vi "CompareData.vi"(1 "Que Name":string, 2 "Data input":string) -> (0 "Same as before":bool)   [LabVIEW 2011]
doc: "Will compare New data with Old Data where the New data is the current Data input and the Old data is the previous Data input."
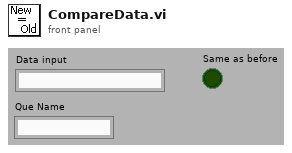
[diagram p1: front panel]
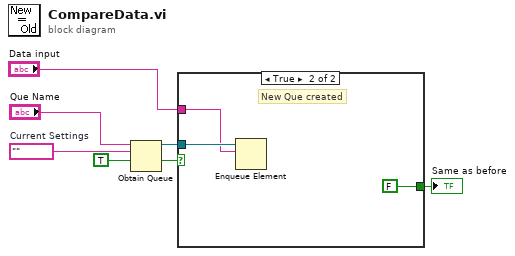
[diagram p0: block diagram]
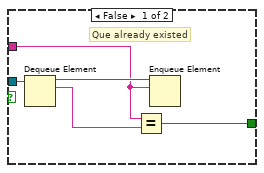
[diagram p2: hidden frame]
diagram:
  w5 = ""  # Current Settings
  n1 = Obtain Queue(name (unnamed)="Que Name", element data type=w5, create if not found? (T)=TRUE) -> (queue out=w6:refnum<queue>, created new?=w4:bool)  [unwired: 2 in, 1 out]
  n2 = case shown="True" w4 {
    tunnel: w6 -> [w12 w15]
    tunnel: "Data input" -> [w9 w14]
    tunnel: [w8 FALSE] -> w2
    frame False {
      # "Que already existed"
      n3 = Dequeue Element(queue=w12) -> (queue out=w11:refnum<queue>, element=w10:string)  [unwired: 2 in, 2 out]
      n4 = Equal?(x=w9, y=w10) -> (x = y?=w8:bool)
      n5 = Enqueue Element(queue=w11, element=w9) -> ()  [unwired: 2 in, 3 out]
    }
    frame True {
      # "New Que created"
      n6 = Enqueue Element(queue=w15, element=w14) -> ()  [unwired: 2 in, 3 out]
    }
  }
  "Same as before" <- w2
